vi "FGV Laser wav min max.vi"(7 "FGV Actions":enum16{"Get", "Set"}(ring), 8 "error in (no error)":errorcluster, 10 "Resp Validated?":bool, 11 "T values":string[](array[string])) -> (0 "error out":errorcluster, 2 "Tmin Out":u16, 3 "Tmax Out":u16)   [LabVIEW 2017]
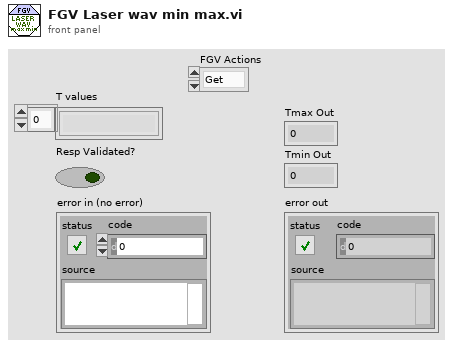
[diagram p1: front panel]
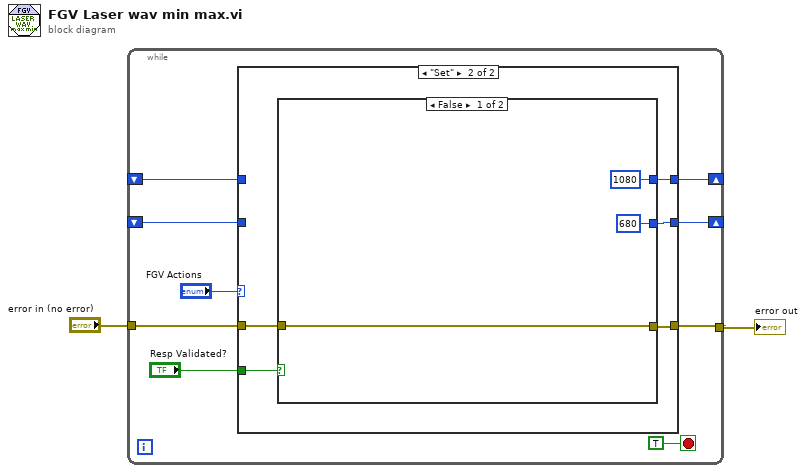
[diagram p0: block diagram]
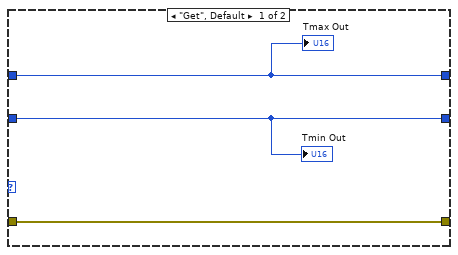
[diagram p2: hidden frame]
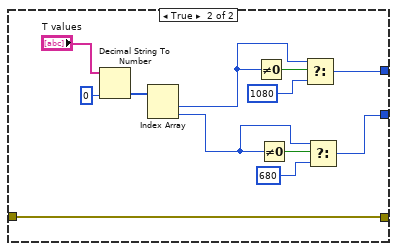
[diagram p3: hidden frame]
diagram:
  n1 = while {
    shift-right: [w9] -> _
    shift-left: _ -> [w8]
    tunnel: "error in (no error)" -> [w7]
    tunnel: [w6] -> w1
    shift-right: [w4] -> _
    shift-left: _ -> [w5]
    stop <- TRUE stop-if-true
    n2 = case shown="\"Set\"" "FGV Actions" {
      tunnel: [w12 w19] -> w9
      tunnel: w8 -> [w12 _]
      tunnel: w7 -> [w14 w16]
      tunnel: [w14 w15] -> w6
      tunnel: w5 -> [w13 _]
      tunnel: [w13 w18] -> w4
      tunnel: "Resp Validated?" -> [_ w17]
      frame "Get", Default {
        "Tmax Out" <- w12
        "Tmin Out" <- w13
      }
      frame "Set" {
        n3 = case shown="False" w17 {
          tunnel: [u16 1080 ("f") w28] -> w19
          tunnel: [u16 680 ("f") w24] -> w18
          tunnel: w16 -> [w22 w23]
          tunnel: [w22 w23] -> w15
          frame False {
          }
          frame True {
            n4 = Decimal String To Number(string="T values", default (0L)=u16 0) -> (number=w33:u16[])  [unwired: 1 in, 1 out]
            n5 = Index Array(array=w33) -> (element #1=w31:u16, element #2=w25:u16)  [unwired: 2 in]
            n6 = Not Equal To 0?(x=w31) -> (x != 0?=w30:bool)
            n7 = Not Equal To 0?(x=w25) -> (x != 0?=w26:bool)
            n8 = Select(t=w31, s=w30, f=u16 1080) -> (s? t:f=w28:u16)
            n9 = Select(t=w25, s=w26, f=u16 680) -> (s? t:f=w24:u16)
          }
        }
      }
    }
  }
  "error out" <- w1
